vi "Config Database_Queue Driver.vi"(8 "error in (no error)":errorcluster, 10 "Enum":T1, 11 "EnQ":string) -> (0 "error out":errorcluster, 3 "DeQ":string)   [LabVIEW 2013, in "ConfigDBLib.lvlib"]
uses:
  ConfigDBLib.lvlib
  Private Controls/Queue Driver Control_Config DB.ctl
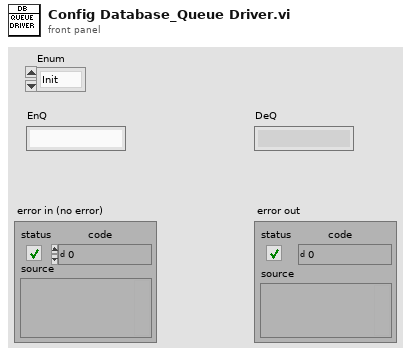
[diagram p1: front panel]
types:
  T1 = typedef "ConfigDBLib.lvlib/Queue Driver Control_Config DB.ctl" = enum16{"Init", "Enqueue", "Dequeue", "ReleaseQueue", "Exit"}
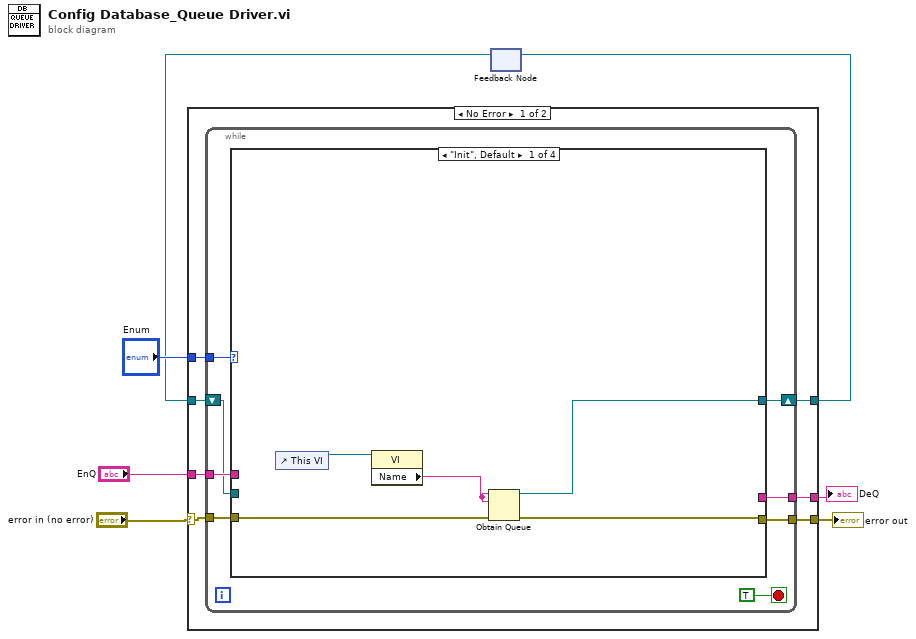
[diagram p0: block diagram]
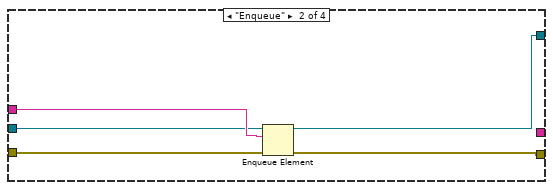
[diagram p2: hidden frame]
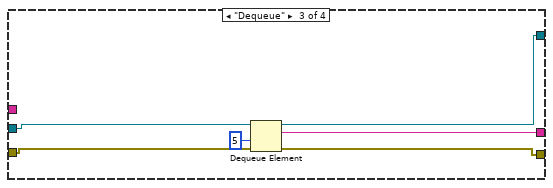
[diagram p3: hidden frame]
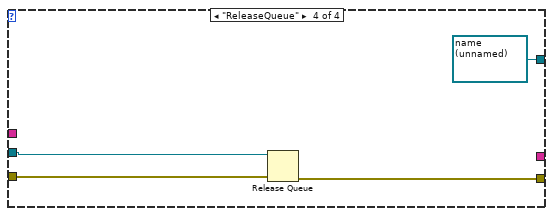
[diagram p4: hidden frame]
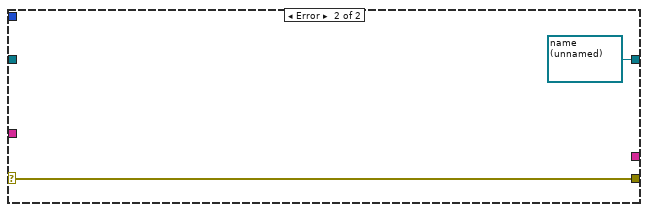
[diagram p5: hidden frame]
diagram:
  n1 = feedback #1() -> (w1:refnum<queue>)  [unwired: 1 in]
  n2 = case shown="No Error" "error in (no error)" {
    selector: "error in (no error)" -> [w12 w44]
    tunnel: [w14 w44] -> w6
    tunnel: "Enum" -> [w13 _]
    tunnel: "EnQ" -> [w11 _]
    tunnel: [w10 _] -> w3
    tunnel: [w9 refnum<queue> refnum ("queue out")] -> w2
    tunnel: w1 -> [w8 _]
    frame No Error {
      n3 = while {
        tunnel: [w22] -> w14
        tunnel: w13 -> [w21]
        shift-right: [w20] -> w9
        shift-left: w8 -> [w17]
        tunnel: w12 -> [w19]
        tunnel: w11 -> [w18]
        tunnel: [w16] -> w10
        stop <- TRUE stop-if-true
        n4 = case shown="\"Init\", Default" w21 {
          tunnel: [w27 w32 w35 w40] -> w22
          tunnel: [w26 w28 w38 refnum<queue> refnum ("queue out")] -> w20
          tunnel: w19 -> [w25 w31 w34 w41]
          tunnel: w18 -> [_ w30 _ _]
          tunnel: w17 -> [_ w29 w37 w42]
          tunnel: [_ _ w36 _] -> w16
          frame "Init", Default {
            n5 = control-ref of="This VI"() -> (w24:refnum<vi>)
            n6 = property class="VI"(reference=w24) -> ("Name"=w23:string)  [unwired: 1 in, 2 out]
            n7 = Obtain Queue(name (unnamed)=w23, element data type=w23, error in (no error)=w25) -> (queue out=w26:refnum<queue>, error out=w27:errorcluster)  [unwired: 2 in, 1 out]
          }
          frame "Enqueue" {
            n8 = Enqueue Element(queue=w29, element=w30, error in (no error)=w31) -> (queue out=w28:refnum<queue>, error out=w32:errorcluster)  [unwired: 1 in, 1 out]
          }
          frame "Dequeue" {
            n9 = Dequeue Element(queue=w37, timeout in ms (-1)=5, error in (no error)=w34) -> (queue out=w38:refnum<queue>, element=w36:string, error out=w35:errorcluster)  [unwired: 1 out]
          }
          frame "ReleaseQueue" {
            n10 = Release Queue(queue=w42, error in (no error)=w41) -> (error out=w40:errorcluster)  [unwired: 1 in, 2 out]
          }
        }
      }
    }
    frame Error {
    }
  }
  "error out" <- w6
  "DeQ" <- w3
  n11 = feedback-in #1(w2) -> ()
